vi "Sensor de temperatura.vi"() -> ()   [LabVIEW 2020]
uses:
  <vilib>/MakerHub/LINX/Public/Peripherals/Digital/Digital Write 1 Chan.vi
  <vilib>/MakerHub/LINX/Public/Peripherals/Analog/Analog Read 1 Chan.vi
  <vilib>/MakerHub/LINX/Public/Peripherals/Digital/Digital Write N Chans.vi
  <vilib>/MakerHub/LINX/Public/Peripherals/Analog/Analog Read N Chans.vi
  <vilib>/MakerHub/LINX/Private/Local IO/LinxDigitalWrite.vi
  <vilib>/MakerHub/LINX/Public/Utilities/Check Channel.vi
  <vilib>/MakerHub/LINX/Private/Local IO/LinxAnalogRead.vi
  <vilib>/MakerHub/LINX/Public/Utilities/Open Serial.vi
  <vilib>/MakerHub/LINX/Private/Utilties/Generate Error.vi
  <vilib>/MakerHub/LINX/LMH-LINX.lvlib
panel:
  in  "LED 3":u8
  in  "Analog Channel":u8
  in  "LED 2":u8
  in  "LED 1":u8
  in  "Serial Port":refnum<visa-resource-name>
  in  "stop":bool
  out "Grados °C":dbl
  out "Frio":bool
  out "Normal":bool
  out "Calor":bool
  out "Variaciones de Temperatura":dbl(graph)
  out "Termometro °C":dbl(slide) scale=0.0..100.0
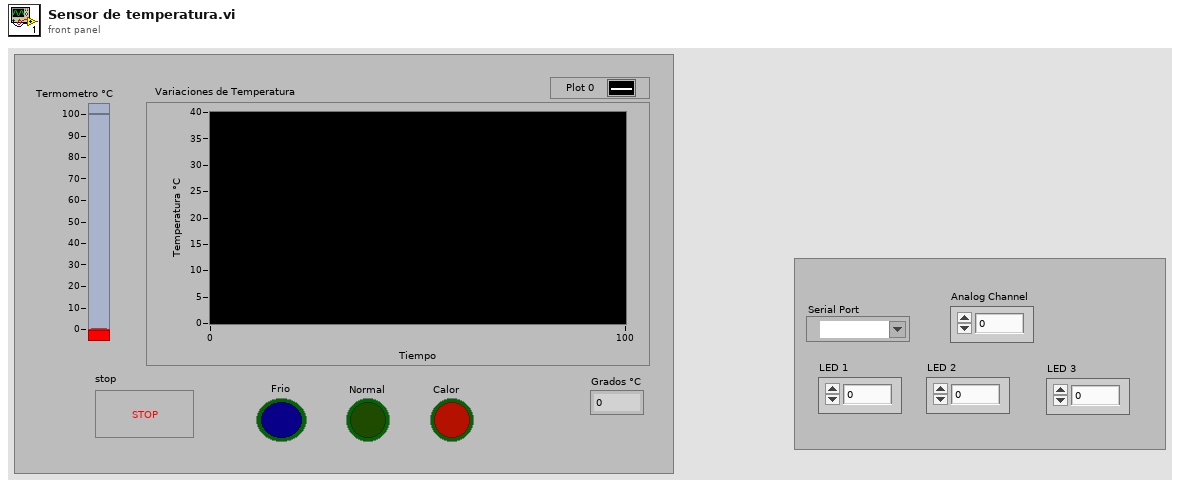
[diagram p1: front panel]
types:
  T1 = typedef "LMH-LINX.lvlib/LINX Ref.ctl" = cluster{"IO":T2, "Interface":T3, "LINX Device Config":T4}
  T2 = typedef "LMH-LINX.lvlib/Platform.ctl" = enum16{"Remote", "Local"}
  T3 = typedef "LMH-LINX.lvlib/Interface.ctl" = enum16{"Serial", "TCP"}
  T4 = typedef "LMH-LINX.lvlib/Device.lvlib/LINX Device Config.ctl" = cluster{"Interface":T3, "COM Port":refnum<visa-resource-name>, "TCP Configuration":T5, "Device Family":u8, "Device ID":u8, "Device Name":string, "TCP Ref":refnum<k5>, "Channels":T6}
  T5 = typedef "LMH-LINX.lvlib/Device.lvlib/TCP Config.ctl" = cluster{"IP Address":string, "Port":u16}
  T6 = typedef "LMH-LINX.lvlib/Channels.ctl" = cluster{"DI":u8[], "DO":u8[], "AI":u8[], "AO":u8[], "PWM":u8[], "QE":u8[], "UART":u8[], "I2C 2":u8[], "SPI":u8[], "CAN":u8[], "Servo":u8[], "AI Ref (V)":dbl, "AI Resolution (Bits)":u8, "AO Ref (V)":dbl, "AO Resolution (Bits)":u8}
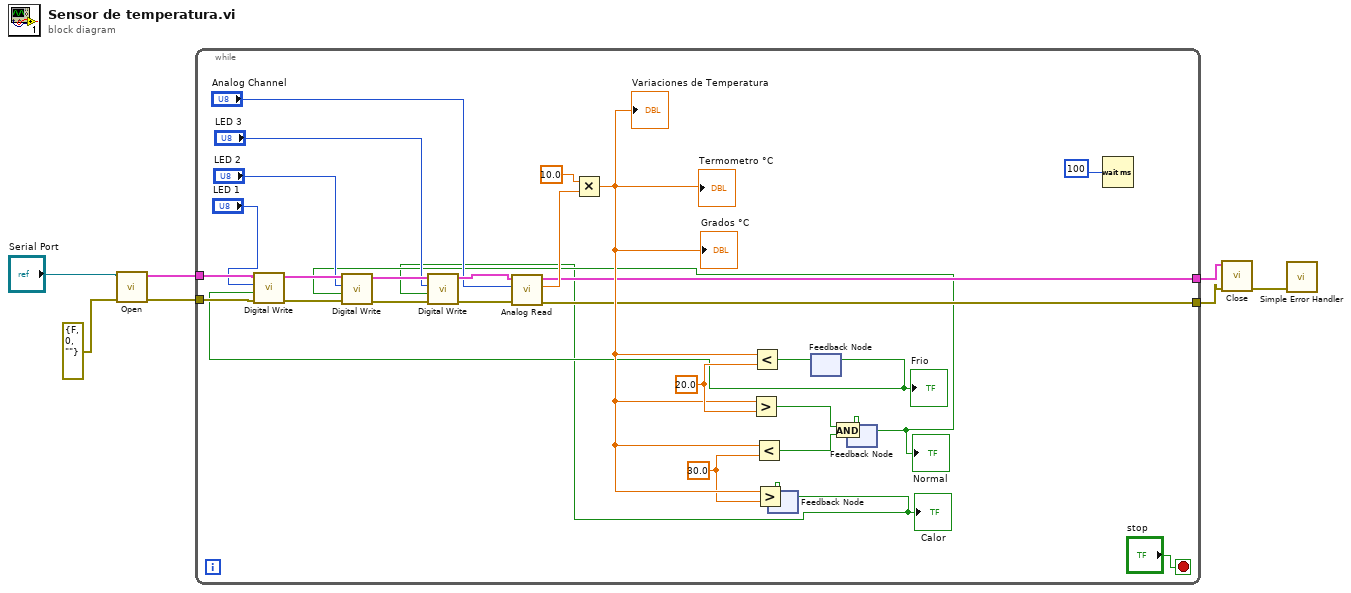
[diagram p0: block diagram]
diagram:
  n1 = call-poly <vilib>:"Open.vi"("Error In"=errorcluster {"status"=FALSE, "code"=0, "source"=""} ("error constant"), "Serial Port"="Serial Port") -> ("Error Out"=w5:errorcluster, "LINX Resource"=w6:T1)  [unwired: 7 in, 1 out]
  n2 = while {
    tunnel: w6 -> [w36]
    tunnel: w5 -> [w35]
    tunnel: [w15] -> w4
    tunnel: [w14] -> w3
    stop <- "stop" stop-if-true
    w20 = 30.0
    w22 = 20.0
    n3 = feedback #1() -> (w8:bool)  [unwired: 1 in]
    "Calor" <- w8
    n4 = feedback #2() -> (w12:bool)  [unwired: 1 in]
    "Frio" <- w12
    n5 = call-poly <vilib>:"Digital Write.vi"("Error In"=w35, "Output Value"=w12, "DO Channel"="LED 1", "LINX Resource"=w36) -> ("Error Out"=w32:errorcluster, "LINX Resource"=w34:T1)  [unwired: 6 in]
    n6 = feedback #3() -> (w10:bool)  [unwired: 1 in]
    "Normal" <- w10
    n7 = call-poly <vilib>:"Digital Write.vi"("Error In"=w32, "Output Value"=w10, "DO Channel"="LED 2", "LINX Resource"=w34) -> ("Error Out"=w31:errorcluster, "LINX Resource"=w33:T1)  [unwired: 6 in]
    n8 = call-poly <vilib>:"Digital Write.vi"("Error In"=w31, "Output Value"=w8, "DO Channel"="LED 3", "LINX Resource"=w33) -> ("Error Out"=w26:errorcluster, "LINX Resource"=w27:T1)  [unwired: 6 in]
    n9 = call-poly <vilib>:"Analog Read.vi"("Error In"=w26, "Analog Channel"="Analog Channel", "LINX Resource"=w27) -> ("Error Out"=w14:errorcluster, "Voltage"=w24:dbl, "LINX Resource"=w15:T1)  [unwired: 5 in, 1 out]
    n10 = Multiply(x=10.0, y=w24) -> (x*y=w21:dbl)
    "Termometro °C" <- w21
    "Variaciones de Temperatura" <- w21
    "Grados °C" <- w21
    n11 = Greater?(x=w21, y=w22) -> (0:w19:bool)
    n12 = Less?(x=w21, y=w22) -> (x < y?=w13:bool)
    n13 = Less?(x=w21, y=w20) -> (x < y?=w18:bool)
    n14 = Greater?(x=w21, y=w20) -> (0:w9:bool)
    n15 = feedback-in #1(w9) -> ()
    n16 = feedback-in #2(w13) -> ()
    n17 = And(x=w19, y=w18) -> (x .and. y?=w11:bool)
    n18 = feedback-in #3(w11) -> ()
    n19 = Wait (ms)(milliseconds to wait=100) -> ()  [unwired: 1 out]
  }
  n20 = call <vilib>:"Close.vi"("Error In"=w3, "LINX Resource"=w4) -> ("Error Out"=w1:errorcluster)  [unwired: 9 in]
  n21 = call <vilib>:"Simple Error Handler.vi"("error in (no error)"=w1) -> ()  [unwired: 4 in, 5 out]
